vi "event structure handling single event.vi"() -> ()   [LabVIEW 2016]
panel:
  in  "Stop":bool
  out "Work done":i32
  out "Iteration number":i32
  in  "Do some work":bool
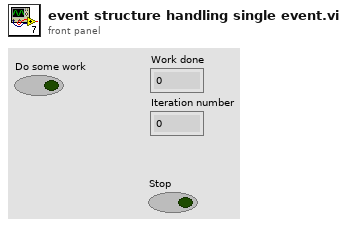
[diagram p1: front panel]
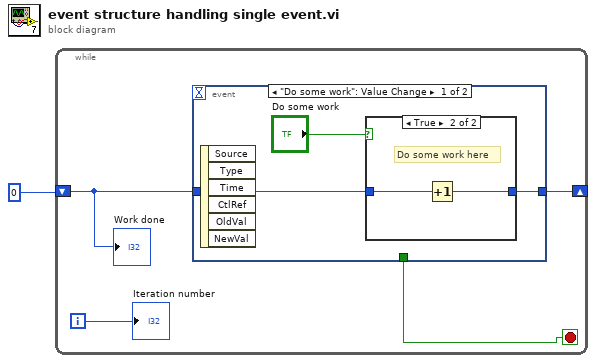
[diagram p0: block diagram]
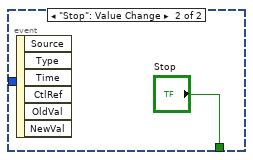
[diagram p3: hidden frame]
diagram:
  n1 = while {
    shift-right: [w5] -> _
    shift-left: 0 -> [w4]
    i -> [w3]
    stop <- w2 stop-if-true
    n2 = event shown="[0] \"Do some work\": Value Change" {
      selector: _ -> [_ _]
      dyn-events: _ -> [_ _]
      timeout: _ -> [_ _]
      tunnel: [w8 _] -> w5
      tunnel: w4 -> [w7 _]
      tunnel: [_ "Stop"] -> w2
      event "Do some work": Value Change {
        n3 = event-data() -> ()  [unwired: 1 in, 6 out]
        n4 = case shown="True" "Do some work" {
          tunnel: w7 -> [w9 w11]
          tunnel: [w9 w10] -> w8
          frame False {
          }
          frame True {
            # "Do some work here"
            n5 = Increment(x=w11) -> (x+1=w10:i32)
          }
        }
      }
      event "Stop": Value Change {
        n6 = event-data() -> ()  [unwired: 1 in, 6 out]
      }
    }
    "Work done" <- w4
    "Iteration number" <- w3
  }
